vi "VRML.vi"(4 "Position":cluster{"X":sgl, "Y":sgl, "Z":sgl}, 8 "error in (no error)":errorcluster, 9 "Path":path, 10 "Name":string) -> (0 "error out":errorcluster, 3 "3D Object out":refnum<class "3D Object.lvclass">)   [LabVIEW 2015, in "3D Object.lvclass"]
uses:
  3D Object.lvclass
  3D Object.lvclass/3D Object.ctl
  <vilib>/picture/3D Picture Control/NI_3D Picture Control.lvlib
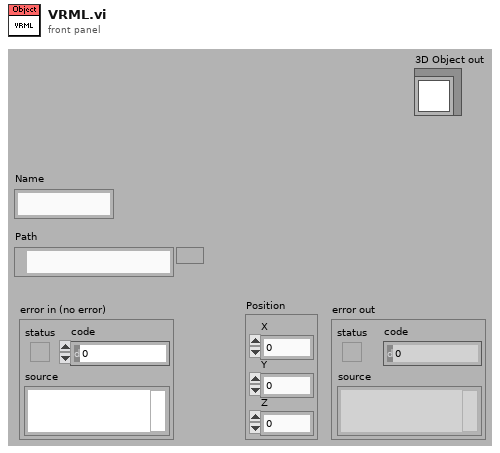
[diagram p1: front panel]
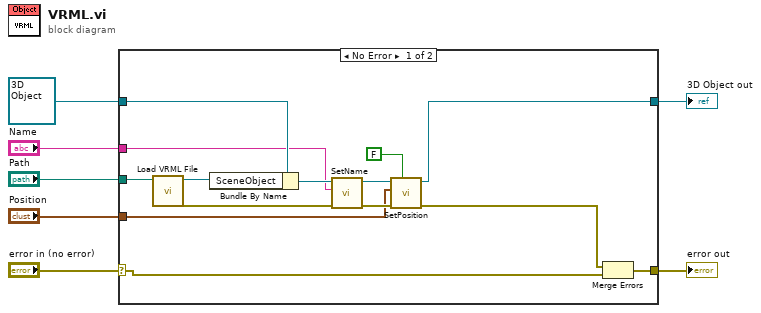
[diagram p0: block diagram]
diagram:
  n1 = case shown="No Error" "error in (no error)" {
    selector: "error in (no error)" -> [w15 w23]
    tunnel: "Path" -> [w21 _]
    tunnel: [w14 w23] -> w6
    tunnel: refnum<class "3D Object.lvclass"> refnum ("3D Object in") -> [w18 w22]
    tunnel: [w9 w22] -> w3
    tunnel: "Name" -> [w17 _]
    tunnel: "Position" -> [w11 _]
    frame No Error {
      n2 = call <vilib>:"Load VRML File.vi"("Path"=w21) -> ("error out"=w16:errorcluster, "Scene:Read Scene File"=w20:refnum<vi>)  [unwired: 1 in, 8 out]
      n3 = Bundle By Name(cluster=w18, "SceneObject"=w20) -> (w19:refnum<class "3D Object.lvclass">)
      n4 = call "SetName.vi"("error in (no error)"=w16, "Name"=w17, "3D Object in"=w19) -> ("error out"=w12:errorcluster, "3D Object out"=w13:refnum<class "3D Object.lvclass">)  [unwired: 7 out]
      n5 = call "SetPosition.vi"("Relative?"=FALSE, "error in (no error)"=w12, "Position"=w11, "3D Object in"=w13) -> ("error out"=w10:errorcluster, "3D Object out"=w9:refnum<class "3D Object.lvclass">)  [unwired: 6 in]
      n6 = Merge Errors(w10, w15) -> (w14:errorcluster)
    }
    frame Error {
    }
  }
  "error out" <- w6
  "3D Object out" <- w3
